vi "Controller Main.vi"() -> ()   [LabVIEW 2011]
uses:
  <vilib>/real-time/rtutility.llb/RT Unlock Target (IP).vi
  <vilib>/real-time/rtutility.llb/RT Lock Target (IP).vi
  <vilib>/rtutility.llb/RT Debug String.vi
  XML VIs/XML Get Actuation Chassis.vi
  XML VIs/XML Get Acquisition Chassis.vi
  <vilib>/Utility/libraryn.llb/Get File Extension.vi
  File VIs/File Read Matrix.vi
  Controller Orbit Correction Matrix Calculation.vi
  File VIs/File Write Matrix.vi
  File VIs/File Read Orbit.vi
  <vilib>/Utility/file.llb/Read From Spreadsheet File.vi
  <vilib>/Utility/file.llb/Read From Spreadsheet File (DBL).vi
  Controller VIs.lvlib
  <vilib>/real-time/NI_Real-Time Libraries.lvlib
  Log VIs.lvlib
  Controller Global Variables.lvlib
  Simulated Beam VIs/Simulated Beam Response.vi
  Simulated Beam VIs.lvlib
  Simulated Beam VIs/Simulated PS Current.vi
panel:
  out "error out":errorcluster
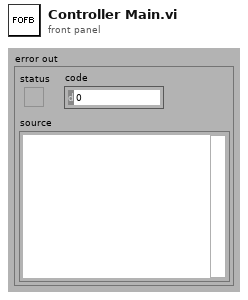
[diagram p1: front panel]
types:
  T1 = enum16{"open", "replace", "create", "open or create", "replace or create", "replace or create with confirmation"}
  T2 = typedef "Type Definitions.lvlib/Type FOFB Configuration.ctl" = cluster{"FOFB Parameters":T3, "Number of Acquisition Chassis":i32, "Number of Actuation Chassis":i32, "Number of BPM Readings":i32, "BPM Reading Names":string[], "Selected BPM Readings":u32[], "Number of Correctors":i32, "Corrector Names":string[], "Selected Correctors":u32[], "Response Matrix":dbl[][][], "Reference Orbit":dbl[][], "Correction Matrix":dbl[][][], "FPGA Filter Sets":cluster{"BPM Filter Coefficients":dbl[][], "PS Filter Coefficients":dbl[][]}[], "Acquisition Chassis Names":string[], "Actuation Chassis Names":string[], "Acquisition Variables":cluster{"Variable Name":string, "Chassis Name":string}[], "Actuation Variables":cluster{"Variable Name":string, "Chassis Name":string}[], "PS Matrix Mapping":cluster{u32[]}[], "Inverse PS Matrix Mapping":u32[][], "BPM Matrix Mapping":cluster{u32[]}[], "Inverse BPM Matrix Mapping":u32[][], "BPM Planes":enum8{"H", "V"}[], "Corrector Planes":enum8{"H", "V"}[]}
  T3 = typedef "Type Definitions.lvlib/Type FOFB Parameters.ctl" = cluster{"Network":T4, "Fast Acquisition":T5, "Acquisition Network":T6, "Actuation Network":T7}
  T4 = typedef "Type Definitions.lvlib/Type Network Configuration.ctl" = cluster{"FOFB Controller IP":string, "LNLS Control Network IP":string, "LNLS Control Network Power Supplies TCP Port":u16, "LNLS Control Network FOFB Configuration TCP Port":u16, "LNLS Control Network BPMs TCP Port":u16, "Monitoring Data TCP Port":u16, "Fast Archiver TCP Port":u16, "Fast Command TCP Port":u16, "TCP Listening Timeout":i32}
  T5 = typedef "Type Definitions.lvlib/Type FA Configuration.ctl" = cluster{"Sampling Period":u32, "Data Buffer Size":u32, "Monitoring Period":u32}
  T6 = typedef "Type Definitions.lvlib/Type Acquisition Network Configuration.ctl" = cluster{"Chassis Name":string, "Variables":cluster{"Variable Name":string, "Matrix Order":u32, "Plane":enum8{"H", "V"}, "On Correction":bool}[]}[]
  T7 = typedef "Type Definitions.lvlib/Type Actuation Network Configuration.ctl" = cluster{"Chassis Name":string, "Variables":cluster{"Variable Name":string, "Matrix Order":u32, "Plane":enum8{"H", "V"}, "On Correction":bool}[]}[]
  T8 = typedef "Type Definitions.lvlib/Type PS Variables.ctl" = cluster{"PS Reading Variables":refnum<k21>[], "PS Setpoint Variables":refnum<k21>[], "PS Status Variables":refnum<k21>[], "PS ON-OFF Variables":refnum<k21>[], "PS Filter Enable":refnum<k21>[], "PS ADDR":refnum<k21>[], "PS DATA":refnum<k21>[]}
  T9 = typedef "Type Definitions.lvlib/Type BPM Variables.ctl" = cluster{"BPM Variables":refnum<k21>[], "BPM Filter Enable":refnum<k21>[], "BPM ADDR":refnum<k21>[], "BPM DATA":refnum<k21>[]}
  T10 = typedef "Type Definitions.lvlib/Type Synchronization Objects.ctl" = cluster{"Blocking":T11, "Non-blocking":T12}
  T11 = typedef "Type Definitions.lvlib/Type Blocking Synchronization Objects.ctl" = cluster{"Monitoring Data Notifier":refnum<notifier>, "Fast Archiver Data FIFO":refnum<queue>, "Operation Mode Change Request FIFO":refnum<k33>, "Monitoring BPM and PS Data FIFO":refnum<k33>, "FA BPM and PS Data FIFO":refnum<k33>, "PS Manual Setpoints FIFO":refnum<k33>, "FOFB Controller Errors FIFO ":refnum<k33>, "FOFB Status In Notifier":refnum<notifier>, "FOFB Status Out Notifier":refnum<notifier>, "PS Configuration Status In Notifier":refnum<notifier>, "PS Configuration Status Out Notifier":refnum<notifier>, "BPM Configuration Status In Notifier":refnum<notifier>, "BPM Configuration Status Out Notifier":refnum<notifier>, "RT Trace Request Queue":refnum<queue>, "Fast Command Data FIFO":refnum<k33>}
  T12 = typedef "Type Definitions.lvlib/Type Non-blocking Synchronization Objects.ctl" = cluster{"FOFB Variables Queue":refnum<queue>, "Diagnostics Data Notifier":refnum<notifier>, "Diagnostics Data (Time-Critical Loop) FIFO":refnum<k33>, "Actuation State Change Request FIFO":refnum<k33>}
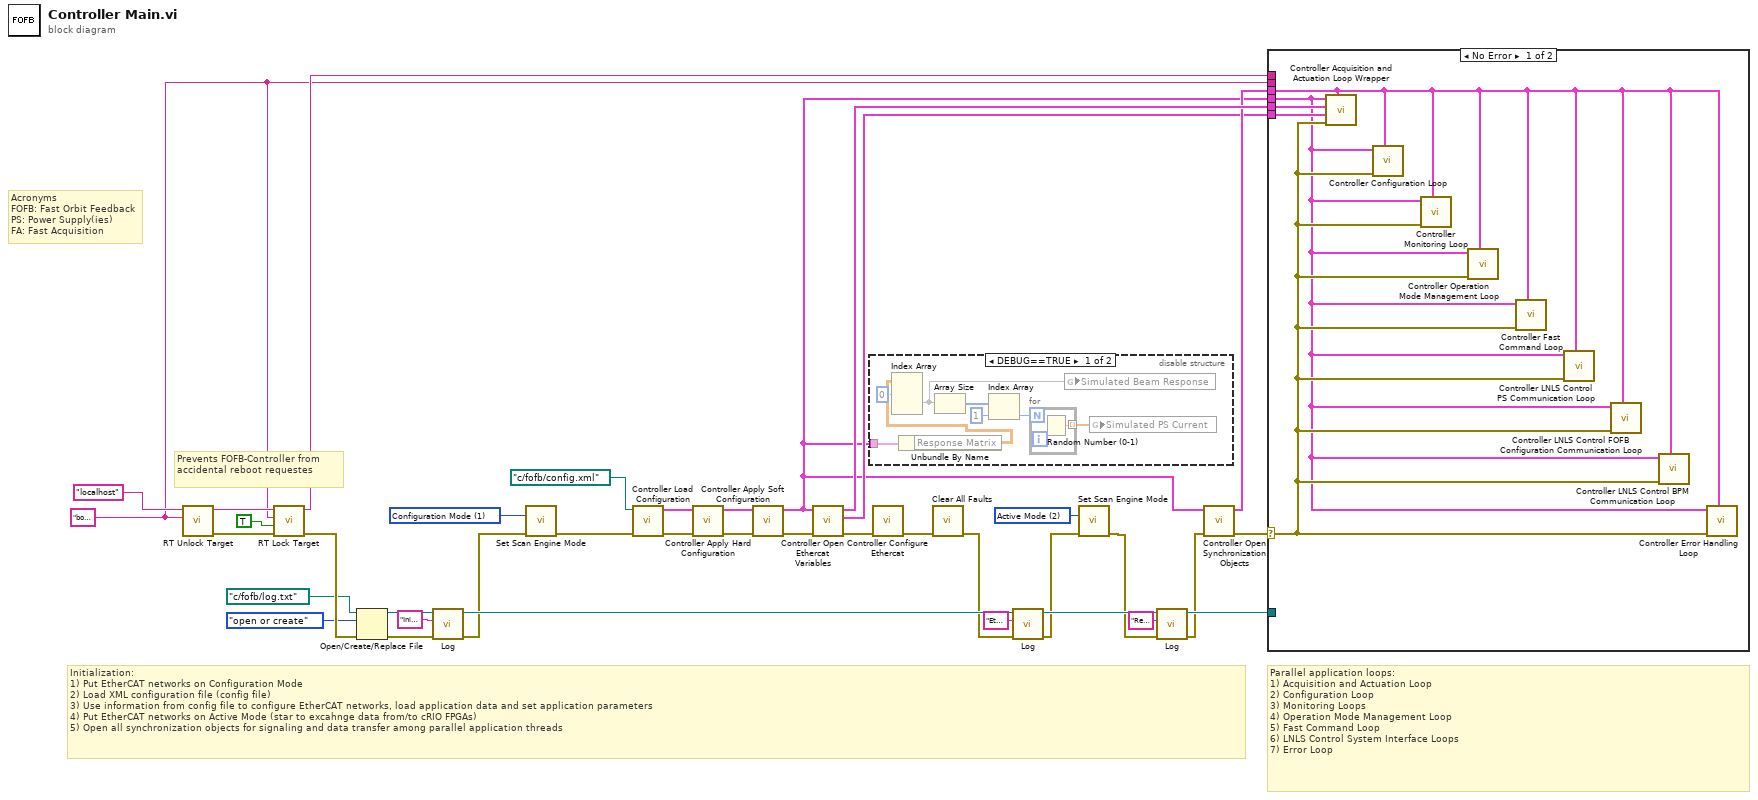
[diagram p0: block diagram]
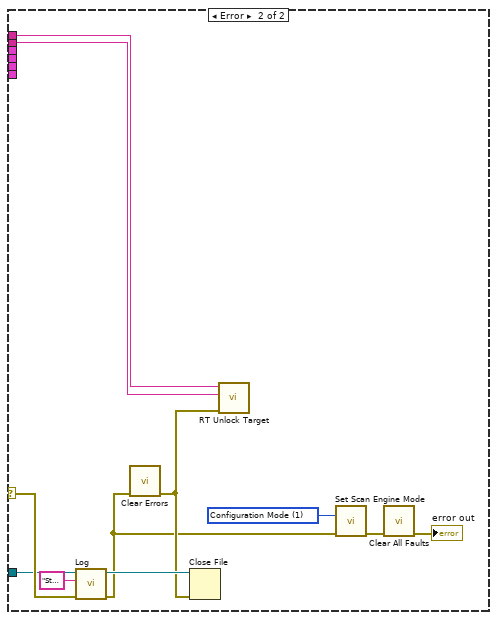
[diagram p3: hidden frame]
diagram:
  w1 = 2 items=["Configuration Mode"=1, "Active Mode"=2] ("mode (Active Mode)")
  w2 = 1 items=["Configuration Mode"=1, "Active Mode"=2] ("mode (Active Mode)")
  w6 = "boo500mev" ("password")
  # "Parallel application loops:\n1) Acquisition and Actuation Loop\n2) Configuration Loop\n3) Monitoring Loops\n4) Operation Mode Management Loop\n5) Fast Command Loop\n6) LNLS Control System Interface Loops\n7) Error Loop"
  # "Initialization:\n1) Put EtherCAT networks on Configuration Mode\n2) Load XML configuration file (config file)\n3) Use information from config file to configure EtherCAT networks, load application data and set application parameters\n4) Put EtherCAT networks on Active Mode (star to excahnge data from/to cRIO FPGAs)\n5) Open all synchronization objects for signaling and data transfer among parallel application threads"
  # "Prevents FOFB-Controller from accidental reboot requestes"
  # "Acronyms\nFOFB: Fast Orbit Feedback\nPS: Power Supply(ies)\nFA: Fast Acquisition"
  n1 = call-poly <vilib>:"RT Unlock Target.vi"("password"=w6, "target address"="localhost") -> ("error out"=w32:errorcluster, "target address out"=w31:string)  [unwired: 7 in, 1 out]
  n2 = call-poly <vilib>:"RT Lock Target.vi"("error in (no error)"=w32, "password-protect restarts? (F)"=TRUE, "password"=w6, "target address"=w31) -> ("error out"=w30:errorcluster, "target address out"=w7:string)  [unwired: 6 in]
  n3 = Open/Create/Replace File(file path (use dialog)=path "c:/fofb/log.txt", error in=w30, operation (0:open)=T1."open or create") -> (refnum out=w27:refnum<file>, error out=w17:errorcluster)  [unwired: 3 in, 1 out]
  n4 = call "Log.vi"("error in (no error)"=w17, "String"="Initializing FOFB-Controller...", "Log File Reference"=w27) -> ("error out"=w15:errorcluster, "Log File Reference"=w20:refnum<file>)  [unwired: 7 in]
  n5 = call <vilib>:"Set Scan Engine Mode.vi"("mode (Active Mode)"=w2, "error in (no error)"=w15) -> ("error out"=w14:errorcluster)  [unwired: 13 in]
  n6 = call "Controller Load Configuration.vi"("error in (no error)"=w14, "FOFB Configuration Path"=path "c:/fofb/config.xml" ("Configuration File Path")) -> ("error out"=w12:errorcluster, "FOFB Configuration"=w10:T2)  [unwired: 8 in]
  n7 = call "Controller Apply Hard Configuration.vi"("error in (no error)"=w12, "FOFB Configuration"=w10) -> ("error out"=w11:errorcluster, "FOFB Configuration"=w9:T2)  [unwired: 8 in]
  n8 = call "Controller Apply Soft Configuration.vi"("error in (no error)"=w11, "FOFB Configuration"=w9) -> ("error out"=w4:errorcluster, "FOFB Configuration"=w3:T2)  [unwired: 8 in]
  n9 = call "Controller Open Ethercat Variables.vi"("error in (no error)"=w4, "FOFB Configuration"=w3) -> ("error out"=w21:errorcluster, "PS Variables"=w34:T8, "BPM Variables"=w37:T9)  [unwired: 7 in]
  n10 = disable-structure shown="DEBUG==TRUE" {
    disable-tunnel: w3 -> [w42 _]
    frame condition #0 {
      n11 = Unbundle By Name(w42) -> ("Response Matrix"=w41:dbl[][][])
      n12 = Index Array(array=w41, index (dim 0)=0 ("index (page)")) -> (element=w40:dbl[][])  [unwired: 2 in]
      n13 = Array Size(array=w40) -> (size(s)=w46:i32[])
      n14 = Index Array(array=w46, index=1) -> (element=w44:i32)
      n15 = for {
        N: w44 -> [_]
        tunnel: [w47] -> w43 mode=indexing
        n16 = Random Number (0-1)() -> (number: 0 to 1=w47:dbl)
      }
      n17 = global write "Simulated Beam Response.vi" "Simulated Beam Response"(w40) -> ()
      n18 = global write "Simulated PS Current.vi" "Simulated PS Current"(w43) -> ()
    }
    frame condition #1 (active) {
    }
  }
  n19 = call "Controller Configure Ethercat.vi"("error in (no error)"=w21) -> ("error out"=w25:errorcluster)  [unwired: 10 in]
  n20 = call <vilib>:"Clear All Faults.vi"("error in (no error)"=w25) -> ("error out"=w19:errorcluster)  [unwired: 1 in, 9 out]
  n21 = call "Log.vi"("error in (no error)"=w19, "String"="EtherCAT acquisition and actuation networks entering in active mode...", "Log File Reference"=w20) -> ("error out"=w18:errorcluster, "Log File Reference"=w22:refnum<file>)  [unwired: 7 in]
  n22 = call <vilib>:"Set Scan Engine Mode.vi"("mode (Active Mode)"=w1, "error in (no error)"=w18) -> ("error out"=w5:errorcluster)  [unwired: 13 in]
  n23 = call "Log.vi"("error in (no error)"=w5, "String"="Reading storage ring status (BPMs and power supplies readings)...", "Log File Reference"=w22) -> ("error out"=w16:errorcluster, "Log File Reference"=w35:refnum<file>)  [unwired: 7 in]
  n24 = call "Controller Open Synchronization Objects.vi"("error in (no error)"=w16, "FOFB Configuration"=w3) -> ("error out"=w38:errorcluster, "Sync Objects"=w36:T10)  [unwired: 8 in]
  n25 = case shown="No Error" w38 {
    selector: w38 -> [w50 w63]
    tunnel: w37 -> [w52 _]
    tunnel: w34 -> [w51 _]
    tunnel: w3 -> [w48 _]
    tunnel: w36 -> [w49 _]
    tunnel: w35 -> [_ w62]
    tunnel: w6 -> [_ w58]
    tunnel: w7 -> [_ w57]
    frame No Error {
      n26 = call "Controller Acquisition and Actuation Loop Wrapper.vi"("Sync Objects"=w49, "error in (no error)"=w50, "PS Variables"=w51, "BPM Variables"=w52, "FOFB Configuration"=w48) -> ()  [unwired: 6 in, 1 out]
      n27 = call "Controller Configuration Loop.vi"("Sync Objects"=w49, "error in (no error)"=w50, "FOFB Configuration"=w48) -> ()  [unwired: 8 in, 1 out]
      n28 = call "Controller Monitoring Loop.vi"("Sync Objects"=w49, "error in (no error)"=w50, "FOFB Configuration"=w48) -> ()  [unwired: 8 in, 1 out]
      n29 = call "Controller Operation Mode Management Loop.vi"("Sync Objects"=w49, "error in (no error)"=w50, "FOFB Configuration"=w48) -> ()  [unwired: 8 in, 1 out]
      n30 = call "Controller Fast Command Loop.vi"("Sync Objects"=w49, "error in (no error)"=w50, "FOFB Configuration"=w48) -> ()  [unwired: 8 in, 1 out]
      n31 = call "Controller LNLS Control PS Communication Loop.vi"("Sync Objects"=w49, "error in (no error)"=w50, "FOFB Configuration"=w48) -> ()  [unwired: 8 in, 1 out]
      n32 = call "Controller LNLS Control FOFB Configuration Communication Loop.vi"("Sync Objects"=w49, "error in (no error)"=w50, "FOFB Configuration"=w48) -> ()  [unwired: 8 in, 1 out]
      n33 = call "Controller LNLS Control BPM Communication Loop.vi"("Sync Objects"=w49, "error in (no error)"=w50, "FOFB Configuration"=w48) -> ()  [unwired: 8 in, 1 out]
      n34 = call "Controller Error Handling Loop.vi"("Sync Objects"=w49, "error in (no error)"=w50, "FOFB Configuration"=w48) -> ()  [unwired: 8 in, 1 out]
    }
    frame Error {
      w53 = 1 items=["Configuration Mode"=1, "Active Mode"=2] ("mode (Active Mode)")
      n35 = call "Log.vi"("error in (no error)"=w63, "String"="Stopping FOFB-Controller...", "Log File Reference"=w62) -> ("error out"=w55:errorcluster, "Log File Reference"=w60:refnum<file>)  [unwired: 7 in]
      n36 = call <vilib>:"Clear Errors.vi"("error in (no error)"=w55) -> ("error out"=w59:errorcluster)  [unwired: 6 in]
      n37 = Close File(refnum=w60, error in=w59) -> ()  [unwired: 2 out]
      n38 = call-poly <vilib>:"RT Unlock Target.vi"("error in (no error)"=w59, "password"=w58, "target address"=w57) -> ()  [unwired: 6 in, 3 out]
      n39 = call <vilib>:"Set Scan Engine Mode.vi"("mode (Active Mode)"=w53, "error in (no error)"=w55) -> ("error out"=w54:errorcluster)  [unwired: 13 in]
      n40 = call <vilib>:"Clear All Faults.vi"("error in (no error)"=w54) -> ("error out"=→"error out":errorcluster)  [unwired: 1 in, 9 out]
    }
  }
